vi "Verify Preconfig.vi"(8 "error in (no error)":errorcluster, 9 "Ref controls":T1, 10 "RED Channel Settings":T2={"Shutter Mode "=2, "Pre-amplifier gain"=1, "Vertical Shift Speed"=0, "Readout Rate "=0, "Exposure Time (s) "=0.0} {"Shutter Mode" items=["Fully Auto", "OPEN", "CLOSED"]}, 11 "Application in":refnum<class "Application.lvclass">) -> (0 "error out":errorcluster, 3 "Application out":refnum<class "Application.lvclass">)   [LabVIEW 2018, in "Application.lvclass"]
doc: "Este VI foi feito para monitorar continuamente a configuração utilizada para o modo de aquisição das câmeras, gerenciando os respectivos indicadores da interface: BIAS, FLAT, COMP ou Read Mode (Fast, Normal ou Slow)."
uses:
  Application.lvclass
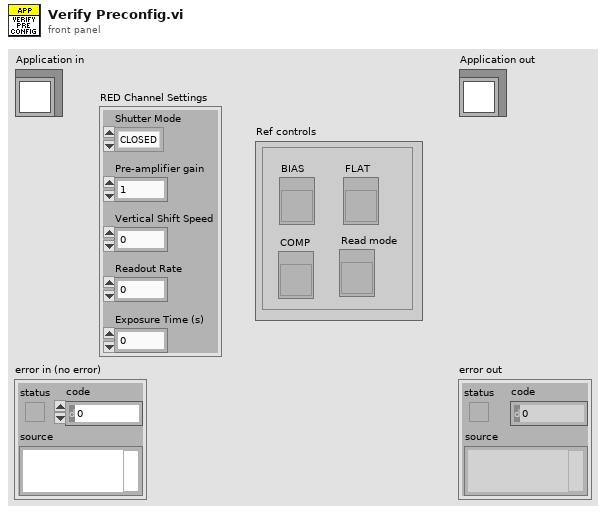
[diagram p1: front panel]
types:
  T1 = cluster{"BIAS":refnum<vi>, "FLAT":refnum<vi>, "COMP":refnum<vi>, "Read mode":refnum<vi>}
  T2 = cluster{"Shutter Mode ":u16, "Pre-amplifier gain":i32, "Vertical Shift Speed":i32, "Readout Rate ":i32, "Exposure Time (s) ":sgl}
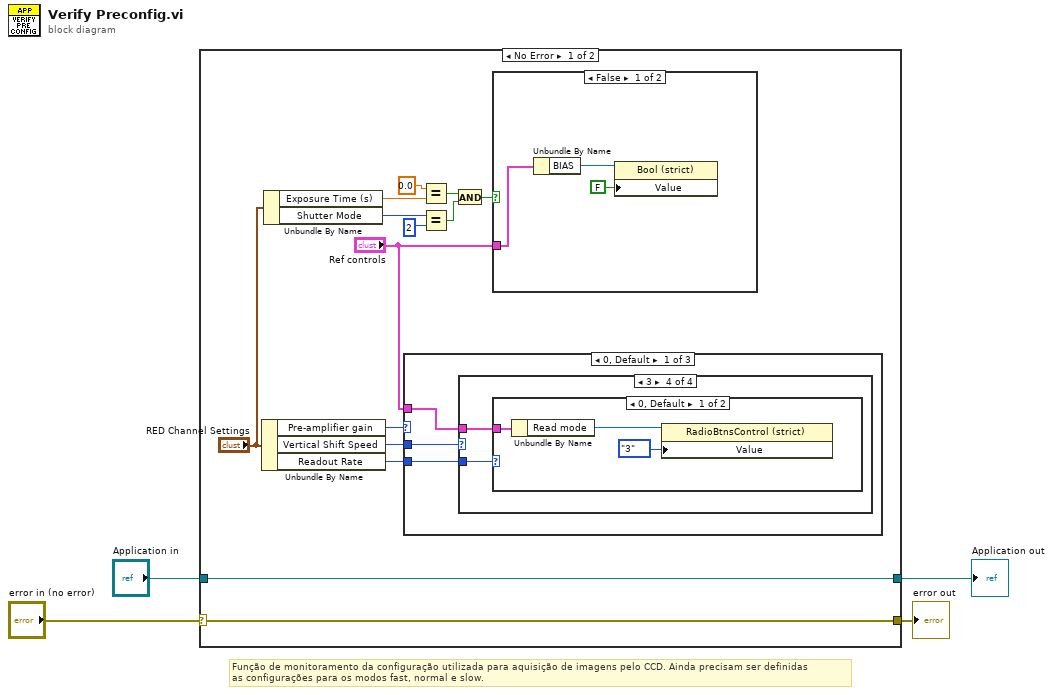
[diagram p0: block diagram]
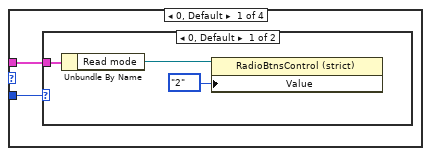
[diagram p2: hidden frame]
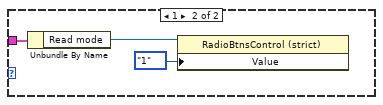
[diagram p3: hidden frame]
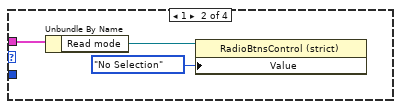
[diagram p4: hidden frame]
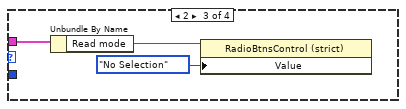
[diagram p5: hidden frame]
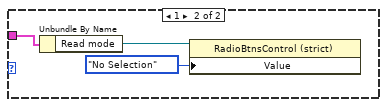
[diagram p6: hidden frame]
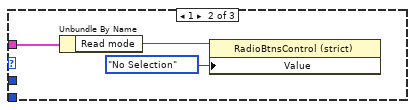
[diagram p7: hidden frame]
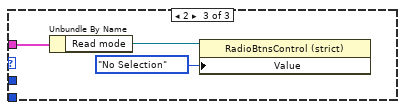
[diagram p8: hidden frame]
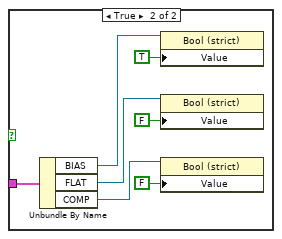
[diagram p9: hidden frame]
diagram:
  # "Função de monitoramento da configuração utilizada para aquisição de imagens pelo CCD. Ainda precisam ser definidas \nas configurações para os modos fast, normal e slow."
  n1 = case shown="No Error" "error in (no error)" {
    selector: "error in (no error)" -> [w10 w61]
    tunnel: [w10 w61] -> w3
    tunnel: [w18 w60] -> w1
    tunnel: "Application in" -> [w18 w60]
    frame No Error {
      n2 = Unbundle By Name("RED Channel Settings") -> ("Pre-amplifier gain"=w8:i32, "Vertical Shift Speed"=w6:i32, "Readout Rate"=w5:i32)
      n3 = Unbundle By Name("RED Channel Settings") -> ("Exposure Time (s)"=w17:sgl, "Shutter Mode"=w15:u16)
      n4 = case shown="0, Default" w8 {
        tunnel: "Ref controls" -> [w21 w44 w47]
        tunnel: w6 -> [w20 _ _]
        tunnel: w5 -> [w19 _ _]
        frame 0, Default {
          n5 = case shown="3" w20 {
            tunnel: w21 -> [w23 w30 w33 w37]
            tunnel: w19 -> [w22 _ _ w36]
            frame 0, Default {
              n6 = case shown="0, Default" w22 {
                tunnel: w23 -> [w24 w29]
                frame 0, Default {
                  n7 = Unbundle By Name(w24) -> ("Read mode"=w26:refnum<vi>)
                  n8 = property class="RadioBtnsControl (strict)"(reference=w26, "Value"=enum32{"No Selection", "1", "2", "3"}."2") -> ()  [unwired: 1 in, 2 out]
                }
                frame 1 {
                  n9 = Unbundle By Name(w29) -> ("Read mode"=w28:refnum<vi>)
                  n10 = property class="RadioBtnsControl (strict)"(reference=w28, "Value"=enum32{"No Selection", "1", "2", "3"}."1") -> ()  [unwired: 1 in, 2 out]
                }
              }
            }
            frame 1 {
              n11 = Unbundle By Name(w30) -> ("Read mode"=w32:refnum<vi>)
              n12 = property class="RadioBtnsControl (strict)"(reference=w32, "Value"=enum32{"No Selection", "1", "2", "3"}."No Selection") -> ()  [unwired: 1 in, 2 out]
            }
            frame 2 {
              n13 = Unbundle By Name(w33) -> ("Read mode"=w35:refnum<vi>)
              n14 = property class="RadioBtnsControl (strict)"(reference=w35, "Value"=enum32{"No Selection", "1", "2", "3"}."No Selection") -> ()  [unwired: 1 in, 2 out]
            }
            frame 3 {
              n15 = case shown="0, Default" w36 {
                tunnel: w37 -> [w40 w41]
                frame 0, Default {
                  n16 = Unbundle By Name(w40) -> ("Read mode"=w39:refnum<vi>)
                  n17 = property class="RadioBtnsControl (strict)"(reference=w39, "Value"=enum32{"No Selection", "1", "2", "3"}."3") -> ()  [unwired: 1 in, 2 out]
                }
                frame 1 {
                  n18 = Unbundle By Name(w41) -> ("Read mode"=w43:refnum<vi>)
                  n19 = property class="RadioBtnsControl (strict)"(reference=w43, "Value"=enum32{"No Selection", "1", "2", "3"}."No Selection") -> ()  [unwired: 1 in, 2 out]
                }
              }
            }
          }
        }
        frame 1 {
          n20 = Unbundle By Name(w44) -> ("Read mode"=w46:refnum<vi>)
          n21 = property class="RadioBtnsControl (strict)"(reference=w46, "Value"=enum32{"No Selection", "1", "2", "3"}."No Selection") -> ()  [unwired: 1 in, 2 out]
        }
        frame 2 {
          n22 = Unbundle By Name(w47) -> ("Read mode"=w49:refnum<vi>)
          n23 = property class="RadioBtnsControl (strict)"(reference=w49, "Value"=enum32{"No Selection", "1", "2", "3"}."No Selection") -> ()  [unwired: 1 in, 2 out]
        }
      }
      n24 = Equal?(x=sgl 0.0, y=w17) -> (x = y?=w12:bool)
      n25 = Equal?(x=w15, y=u16 2) -> (x = y?=w13:bool)
      n26 = And(x=w12, y=w13) -> (x .and. y?=w11:bool)
      n27 = case shown="False" w11 {
        tunnel: "Ref controls" -> [w52 w59]
        frame False {
          n28 = Unbundle By Name(w52) -> ("BIAS"=w51:refnum<vi>)
          n29 = property class="Bool (strict)"(reference=w51, "Value"=FALSE) -> ()  [unwired: 1 in, 2 out]
        }
        frame True {
          n30 = Unbundle By Name(w59) -> ("BIAS"=w58:refnum<vi>, "FLAT"=w56:refnum<vi>, "COMP"=w55:refnum<vi>)
          n31 = property class="Bool (strict)"(reference=w58, "Value"=TRUE) -> ()  [unwired: 1 in, 2 out]
          n32 = property class="Bool (strict)"(reference=w56, "Value"=FALSE) -> ()  [unwired: 1 in, 2 out]
          n33 = property class="Bool (strict)"(reference=w55, "Value"=FALSE) -> ()  [unwired: 1 in, 2 out]
        }
      }
    }
    frame Error {
    }
  }
  "error out" <- w3
  "Application out" <- w1
